vi "Menu Button - Value Change.vi"(7 "RadioButtonsControl in":refnum<vi>, 9 "Numeric":i32, 10 "Display State In in":T2={"Header"="", "Label[]"=[], "DisableButtonsLUT"=variant(string[] []), "Menu Config"=variant}, 11 "Data In in":T1) -> (2 "Display State In out":T2={"Header"="", "Label[]"=[], "DisableButtonsLUT"=variant(string[] []), "Menu Config"=variant}, 3 "Data In out":T1)   [LabVIEW 2019, in "Menu Button.xctl"]
doc: "JSMA Module Template - Top Level UI 0.2.0.4\nRob Humfeld - Jet Engineering\nCopyright (c) 2019, Jet Engineering"
uses:
  Menu Button.xctl
  State 1.ctl
  Data 1.ctl
  Button Config Cluster STYP.ctl
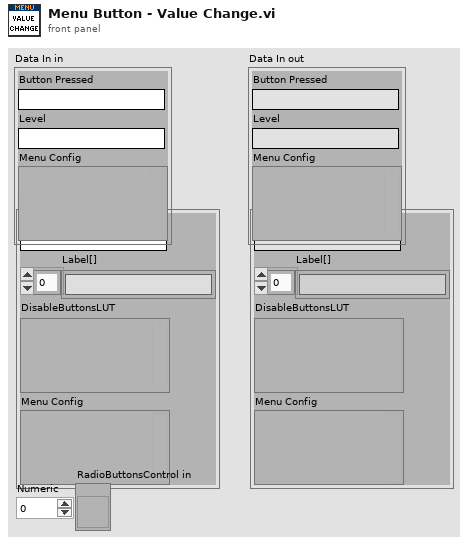
[diagram p1: front panel]
types:
  T1 = typedef "Menu Button.xctl/Data 1.ctl" = cluster{"Button Pressed":string, "Level":string, "Menu Config":variant}
  T2 = typedef "Menu Button.xctl/State 1.ctl" = cluster{"Header":string, "Label[]":string[], "DisableButtonsLUT":variant, "Menu Config":variant}
  T3 = enum32{"No Selection", "System Setup", "System Monitor", "Test Selection", "Data Review", "Radio Selection 5", "Radio Selection 6", "Radio Selection 7", "Radio Selection 8", "Radio Selection 9", "Radio Selection 10"}
  T4 = typedef "Menu Button.xctl/Button Config Cluster STYP.ctl" = cluster{"ID":string, "Name":string, "Action":string, "Value":string, "Enable?":bool, "Color":string}
  T5 = typedef "Menu Button.xctl/Level Config Cluster STYP.ctl" = cluster{"ID":string, "Label":string, "Button.ID[]":string[]}
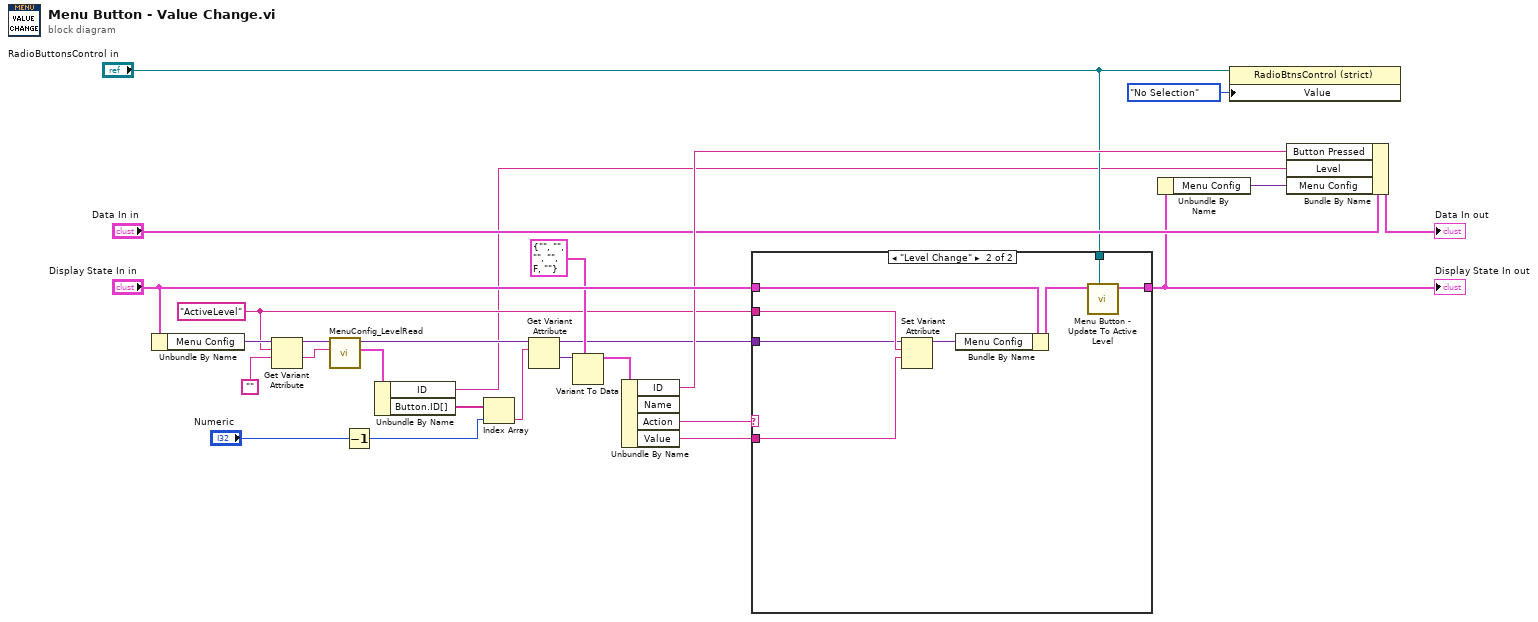
[diagram p0: block diagram]
diagram:
  w13 = "ActiveLevel" ("name")
  n1 = Unbundle By Name("Display State In in") -> ("Menu Config"=w18:variant)
  n2 = Get Variant Attribute(Variant=w18, name=w13, default value (empty Variant)="") -> (duplicate Variant=w5:variant, value=w6:string)  [unwired: 1 in, 2 out]
  n3 = call "MenuConfig_LevelRead.vi"("Level.ID"=w6, "MenuConfig"=w5) -> ("LevelConfig"=w4:T5, "MenuConfig"=w2:variant)  [unwired: 7 in, 1 out]
  n4 = Decrement(x="Numeric") -> (x-1=w12:i32)
  n5 = Unbundle By Name(w4) -> ("ID"=w1:string, "Button.ID[]"=w3:string[])
  n6 = Index Array(array=w3, index=w12) -> (element=w20:string)
  n7 = Get Variant Attribute(Variant=w2, name=w20) -> (duplicate Variant=w14:variant, value=w21:variant)  [unwired: 2 in, 2 out]
  n8 = Variant To Data(type=T4 {"ID"="", "Name"="", "Action"="", "Value"="", "Enable?"=FALSE, "Color"=""} ("ButtonConfig"), Variant=w21) -> (data=w15:T4)  [unwired: 1 in, 1 out]
  n9 = Unbundle By Name(w15) -> ("ID"=w24:string, "Action"=w25:string, "Value"=w16:string)  [unwired: 1 out]
  n10 = case shown="\"Level Change\"" w25 {
    tunnel: "Display State In in" -> [w27 w35]
    tunnel: [w27 w32] -> w9
    tunnel: w16 -> [_ w28]
    tunnel: w14 -> [_ w29]
    tunnel: w13 -> [_ w30]
    tunnel: "RadioButtonsControl in" -> [_ w31]
    frame Default {
    }
    frame "Level Change" {
      n11 = Set Variant Attribute(Variant=w29, name=w30, value=w28) -> (Variant out=w34:variant)  [unwired: 1 in, 2 out]
      n12 = Bundle By Name(cluster=w35, "Menu Config"=w34) -> (w33:T2)
      n13 = call "Menu Button - Update To Active Level.vi"("RadioButtonsControl in"=w31, "Display State In in"=w33) -> ("Display State In out"=w32:T2)  [unwired: 9 in]
    }
  }
  "Display State In out" <- w9
  n14 = Unbundle By Name(w9) -> ("Menu Config"=w8:variant)
  n15 = property class="RadioBtnsControl (strict)"(reference="RadioButtonsControl in", "Value"=T3."No Selection") -> ()  [unwired: 1 in, 2 out]
  n16 = Bundle By Name(cluster="Data In in", "Button Pressed"=w24, "Level"=w1, "Menu Config"=w8) -> (→"Data In out":T1)
